vi "Test.vi"() -> ()   [LabVIEW 2011]
panel:
  in  "Boolean 2":bool
  out "Boolean":bool
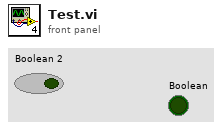
[diagram p1: front panel]
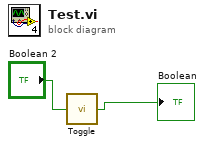
[diagram p0: block diagram]
diagram:
  n1 = call "Toggle.vi"("Input Control"="Boolean 2") -> ("Status"=→"Boolean":bool)
